vi "读取初始位置.vi"() -> (2 "PosOut":dbl[](array[numeric]) caption="第一行")   [LabVIEW 2018]
uses:
  <vilib>/Utility/file.llb/Read Delimited Spreadsheet (DBL).vi
panel:
  in  "请选择标定文件":path
  in  "取消":bool
  in  "确定":bool
  # "选择使用Alligent.exe标定好的位置文件，否则会采用默认位置，可能导致测量失败"
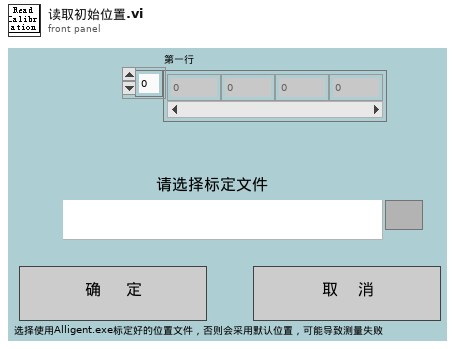
[diagram p1: front panel]
types:
  T1 = enum8{"Enabled", "Disabled", "Disabled and Grayed Out"}
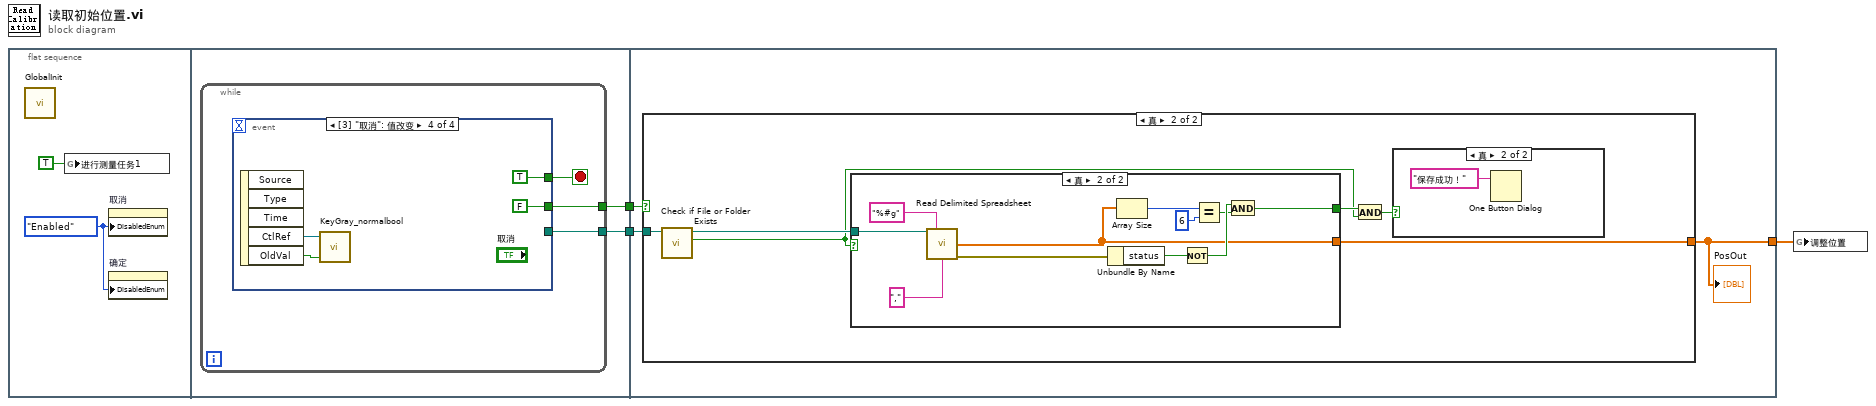
[diagram p0: block diagram]
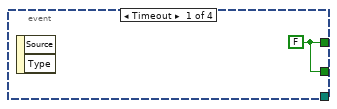
[diagram p2: hidden frame]
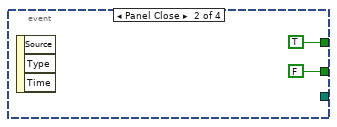
[diagram p3: hidden frame]
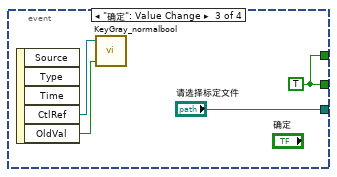
[diagram p4: hidden frame]
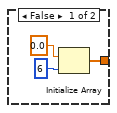
[diagram p5: hidden frame]
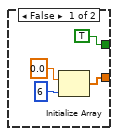
[diagram p6: hidden frame]
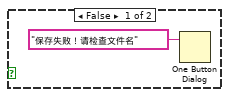
[diagram p7: hidden frame]
diagram:
  n1 = flat-sequence {
    tunnel: [w7] -> w3
    tunnel: [w6] -> w2
    tunnel: w3 -> [w24]
    tunnel: w2 -> [w23]
    tunnel: [w22] -> w1
    frame #0 {
      w5 = T1."Enabled" ("禁用")
      n2 = call "GlobalInit.vi"() -> ()  [unwired: 1 in, 1 out]
      n3 = global write "参数.vi" "进行测量任务1"(TRUE ("是否完成本次测量？")) -> ()
      n4 = property on="取消" class="Bool (严格)"("DisabledEnum"=w5) -> ()  [unwired: 2 in, 2 out]
      n5 = property on="确定" class="Bool (严格)"("DisabledEnum"=w5) -> ()  [unwired: 2 in, 2 out]
    }
    frame #1 {
      n6 = while {
        tunnel: [w9] -> w6
        tunnel: [w8] -> w7
        stop <- w10 stop-if-true
        n7 = event shown="[3] \"取消\": 值改变" {
          selector: _ -> [_ _ _ _]
          dyn-events: _ -> [_ _ _ _]
          timeout: _ -> [_ _ _ _]
          tunnel: [w11 TRUE w15 TRUE] -> w10
          tunnel: [w11 FALSE w15 FALSE] -> w9
          tunnel: [_ _ "请选择标定文件" _] -> w8
          event Timeout {
            w11 = FALSE
            n8 = event-data() -> ()  [unwired: 1 in, 2 out]
          }
          event Panel Close {
            n9 = event-data() -> ()  [unwired: 1 in, 3 out]
          }
          event "确定": Value Change {
            w15 = TRUE
            n10 = event-data() -> ("CtlRef"=w17:refnum<vi>, "OldVal"=w16:bool)  [unwired: 1 in, 3 out]
            n11 = call "KeyGray_normalbool.vi"("OldVal"=w16, "引用"=w17) -> ()  [unwired: 2 in]
          }
          event "取消": Value Change {
            n12 = event-data() -> ("CtlRef"=w20:refnum<vi>, "OldVal"=w19:bool)  [unwired: 1 in, 3 out]
            n13 = call "KeyGray_normalbool.vi"("OldVal"=w19, "引用"=w20) -> ()  [unwired: 2 in]
          }
        }
      }
    }
    frame #2 {
      n14 = case shown="真" w23 {
        tunnel: w24 -> [_ w33]
        tunnel: [w25 w28] -> w22
        frame False {
          n15 = Initialize Array(0.0, 6 ("维数大小")) -> (w25:dbl[])
        }
        frame True {
          n16 = call <vilib>:"Check if File or Folder Exists.vi"("path"=w33) -> ("file or folder exists?"=w30:bool, "dup path"=w32:path)  [unwired: 8 in, 1 out]
          n17 = case shown="真" w30 {
            tunnel: w32 -> [_ w48]
            tunnel: [TRUE w39] -> w31
            tunnel: [w34 w38] -> w28
            frame False {
              n18 = Initialize Array(0.0, 6 ("维数大小")) -> (w34:dbl[])
            }
            frame True {
              n19 = call-poly <vilib>:"Read Delimited Spreadsheet.vi"("file path (dialog if empty)"=w48, "format (%.3f)"="%#g", "delimiter (\\t)"="," ("delimiter (\\t)")) -> ("first row"=w38:dbl[], "error out"=w45:errorcluster)  [unwired: 7 in, 4 out]
              n20 = Unbundle By Name(w45) -> ("status"=w44:bool)
              n21 = Array Size(array=w38) -> (size(s)=w43:i32)
              n22 = Not(x=w44) -> (.not. x?=w41:bool)
              n23 = Equal?(x=w43, y=6) -> (x = y?=w40:bool)
              n24 = And(x=w41, y=w40) -> (x .and. y?=w39:bool)
            }
          }
          n25 = And(x=w31, y=w30) -> (x .and. y?=w29:bool)
          n26 = case shown="真" w29 {
            frame False {
              n27 = One Button Dialog(message="保存失败！请检查文件名" ("消息")) -> ()  [unwired: 1 in, 1 out]
            }
            frame True {
              n28 = One Button Dialog(message="保存成功！" ("消息")) -> ()  [unwired: 1 in, 1 out]
            }
          }
        }
      }
      "PosOut" <- w22
    }
  }
  n29 = global write "globalMessage.vi" "调整位置"(w1) -> ()
